vi "Configuration.vi"(6 "Return Data":refnum<user-event>, 8 "error in (no error)":errorcluster, 9 "Exit Running Config":refnum<user-event>, 10 "Panel in":refnum<class "Panel.lvclass">, 11 "No Popup Data Type in":refnum<class "No Popup Data Type.lvclass">) -> (0 "error out":errorcluster, 3 "No Popup Data Type out":refnum<class "No Popup Data Type.lvclass">)   [LabVIEW 2018, in "No Popup Data Type.lvclass"]
uses:
  No Popup Data Type.lvclass
  D:/Code/QControls Extended/DataGrid/DataGrid Configuration/Data Type Classes/Generic/Generic Data Type.lvclass
  <vilib>/MGI/Panel Manager/Panel/Panel/Panel.lvclass
  Generic/Generic Data Type.lvclass
  Generic/Generic Data Type.lvclass/Generic Data Type.ctl
  Generic/Write Column Header.vi
  Generic/Read Column Header.vi
panel:
  in  "Column Header":string
  # "Non-Editable Column"
  # "This column will be uneditable."
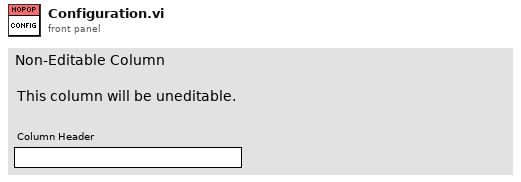
[diagram p1: front panel]
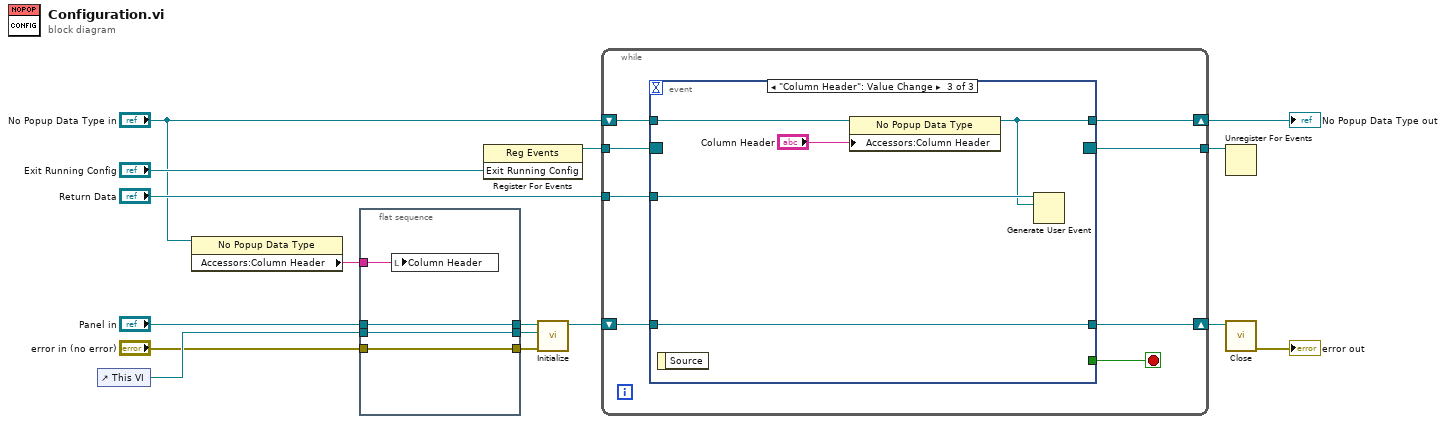
[diagram p0: block diagram]
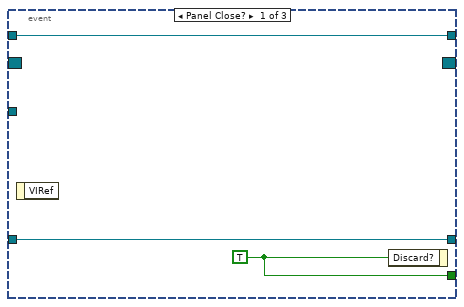
[diagram p2: hidden frame]
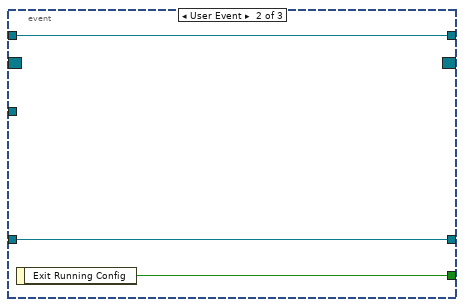
[diagram p3: hidden frame]
diagram:
  n1 = control-ref of="This VI"() -> (w6:refnum<vi>)
  n2 = property class="No Popup Data Type"(reference="No Popup Data Type in") -> ("Accessors:Column Header"=w1:string)  [unwired: 1 in, 2 out]
  n3 = flat-sequence {
    tunnel: [w20] -> w9
    tunnel: "Panel in" -> [w20]
    tunnel: [w19] -> w7
    tunnel: w6 -> [w19]
    tunnel: "error in (no error)" -> [w18]
    tunnel: [w18] -> w4
    tunnel: w1 -> [w17]
    frame #0 {
      n4 = local write "Column Header"(w17) -> ()
    }
  }
  n5 = register-events("Exit Running Config") -> (reference out=w16:refnum<event-registration>)  [unwired: 2 in, 1 out]
  n6 = call <vilib>:"Initialize.vi"("error in (no error)"=w4, "VI Refnum"=w7, "Panel In"=w9) -> ("Panel Out"=w14:refnum<class "Panel.lvclass">)  [unwired: 6 in, 2 out]
  n7 = while {
    shift-right: [w22] -> w11
    shift-left: "No Popup Data Type in" -> [w28]
    shift-right: [w24] -> w12
    shift-left: w14 -> [w25]
    tunnel: w16 -> [w26]
    tunnel: [w23] -> w13
    tunnel: "Return Data" -> [w21]
    stop <- w27 stop-if-true
    n8 = event shown="[2] \"Column Header\": Value Change" {
      selector: w26 -> [_ _ _]
      dyn-events: [_ _ _] -> w23
      timeout: _ -> [_ _ _]
      tunnel: w28 -> [w31 w34 w39]
      tunnel: [w31 w34 w35] -> w22
      tunnel: [w30 w32 _] -> w27
      tunnel: w25 -> [w29 w33 w37]
      tunnel: [w29 w33 w37] -> w24
      tunnel: w21 -> [_ _ w36]
      event Panel Close? {
        w30 = TRUE
        n9 = event-data() -> ()  [unwired: 1 in, 1 out]
        n10 = event-data("Discard?"=w30) -> ()  [unwired: 1 in, 1 out]
      }
      event User Event {
        n11 = event-data() -> ("Exit Running Config"=w32:bool)  [unwired: 1 in]
      }
      event "Column Header": Value Change {
        n12 = event-data() -> ()  [unwired: 1 in, 1 out]
        n13 = property class="No Popup Data Type"(reference=w39, "Accessors:Column Header"="Column Header") -> (reference out=w35:refnum<class "No Popup Data Type.lvclass">)  [unwired: 1 in, 1 out]
        n14 = Generate User Event(user event=w36, event data cluster=w35) -> ()  [unwired: 2 in, 2 out]
      }
    }
  }
  "No Popup Data Type out" <- w11
  n15 = Unregister For Events(event registration refnum=w13) -> ()  [unwired: 1 in, 1 out]
  n16 = call-dynamic "Close.vi"("Panel In"=w12) -> ("Error Out"=→"error out":errorcluster)  [unwired: 10 in]
